vi "Configure Reading Format of Display.vi"(8 "error in (no error)":errorcluster, 10 "Reading Format (0: Exponent)":u16(ring) items=["Exponent", "Prefix"], 11 "VISA resource name":refnum<visa-resource-name>) -> (0 "error out":errorcluster, 3 "VISA resource name out":refnum<visa-resource-name>)   [LabVIEW 2022 SP3, in "Keithley 2450.lvlib"]
doc: "This VI sets the format that is used to display measurement readings on the front-panel display of\nthe instrument. Prefix or Exponent format."
uses:
  Keithley 2450.lvlib
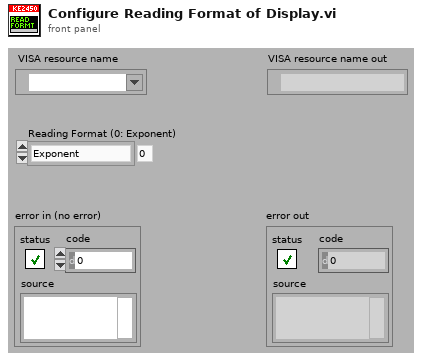
[diagram p1: front panel]
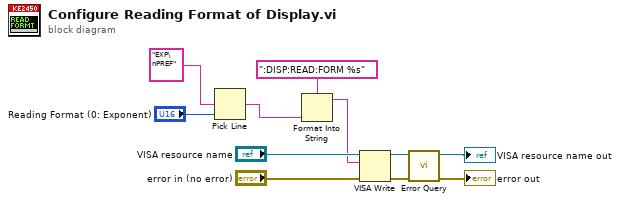
[diagram p0: block diagram]
diagram:
  n1 = Pick Line(multi-line string="EXP\nPREF", line index="Reading Format (0: Exponent)") -> (output string=w1:string)  [unwired: 1 in]
  n2 = Format Into String(format string=":DISP:READ:FORM %s", w1) -> (resulting string=w4:string)  [unwired: 2 in, 1 out]
  n3 = VISA Write(VISA resource name="VISA resource name", write buffer=w4, error in (no error)="error in (no error)") -> (VISA resource name out=w9:refnum<visa-resource-name>, error out=w6:errorcluster)  [unwired: 1 out]
  n4 = call "Error Query.vi"("error in (no error)"=w6, "VISA resource name"=w9) -> ("error out"=→"error out":errorcluster, "VISA resource name out"=→"VISA resource name out":refnum<visa-resource-name>)  [unwired: 8 out]
